vi "Read file.vi"(5 "Clk index":i32=1, 7 "Det index":i32, 8 "error in (no error)":errorcluster, 10 "Averaging range":dbl=1e-08 format="%#_13g", 11 "file (use dialog) in":path) -> (0 "Error Out":errorcluster, 1 "Polarity":enum16{"falling", "rising"}(ring), 2 "Waveform Array":waveform(dbl)[](array[waveform]), 3 "file (use dialog) out":path)   [LabVIEW 2020]
uses:
  <vilib>/Analysis/baseanly.llb/Mean (DBL).vi
  <vilib>/Utility/xml.llb/Read From XML File(array).vi
  <vilib>/Analysis/NI_AALBase.lvlib
panel:
  out "Running average (use odd integer)":i32=9
  out "XML Elements":string[](array[string])
  out "dt":dbl[](array[numeric])
  out "Ys":dbl[][](array[numeric])
  out "before substring":string
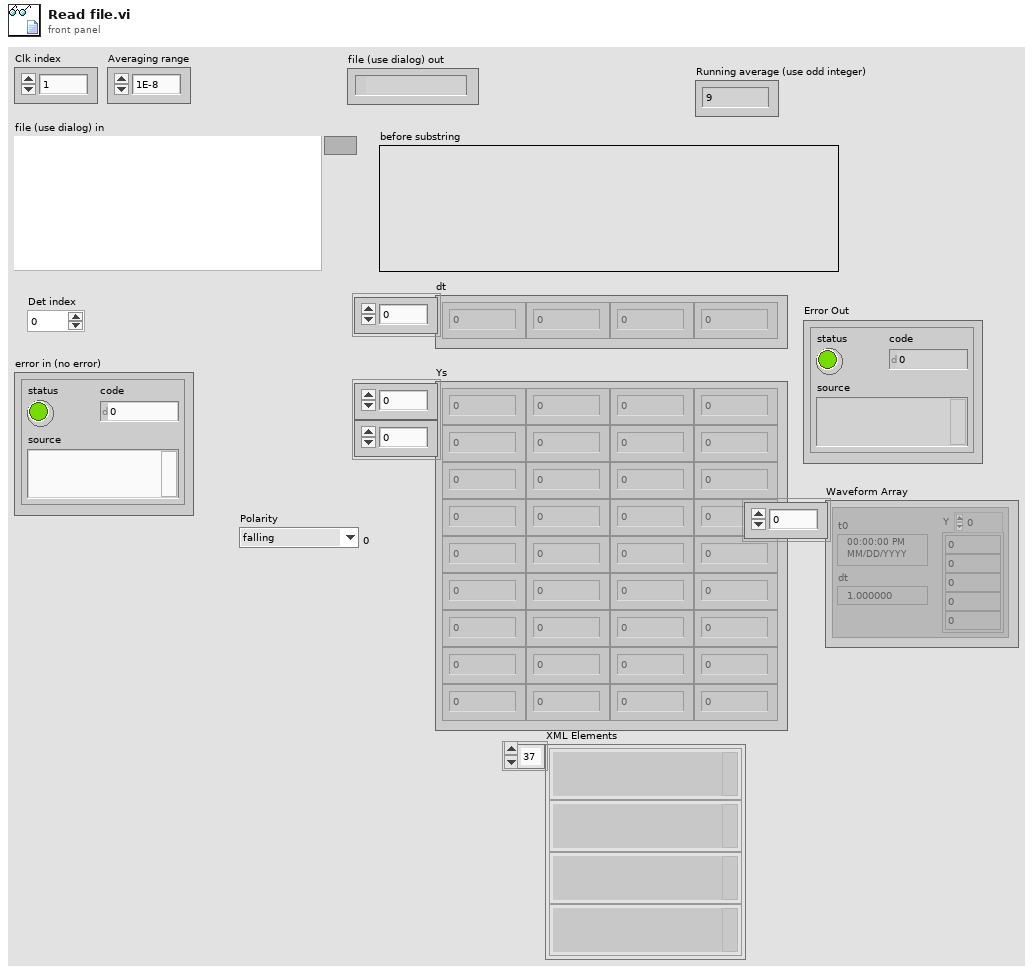
[diagram p1: front panel]
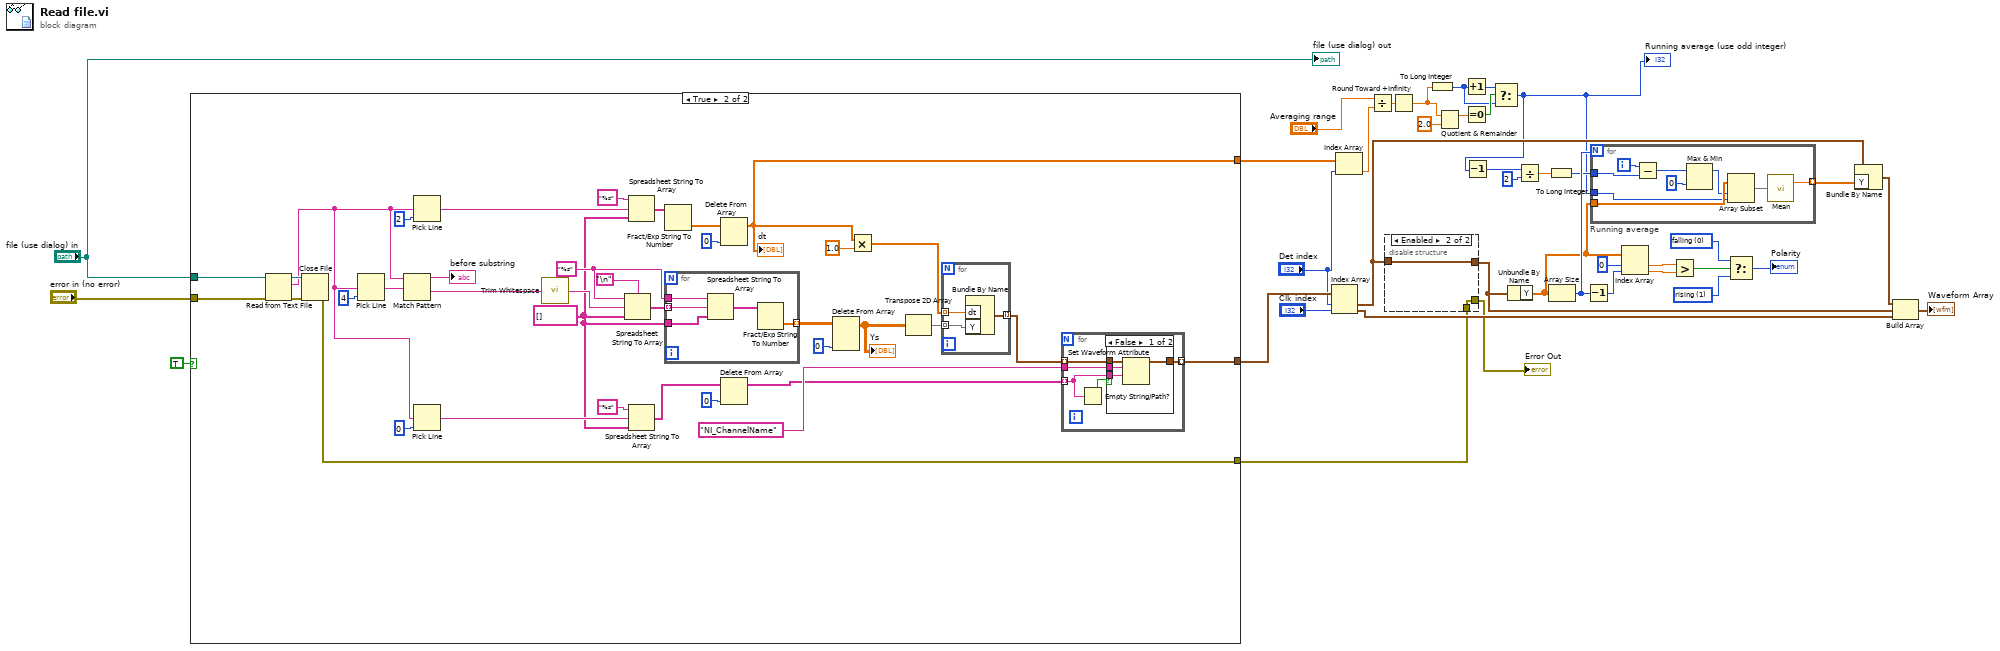
[diagram p0: block diagram]
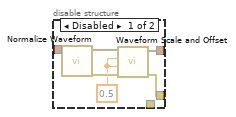
[diagram p2: hidden frame]
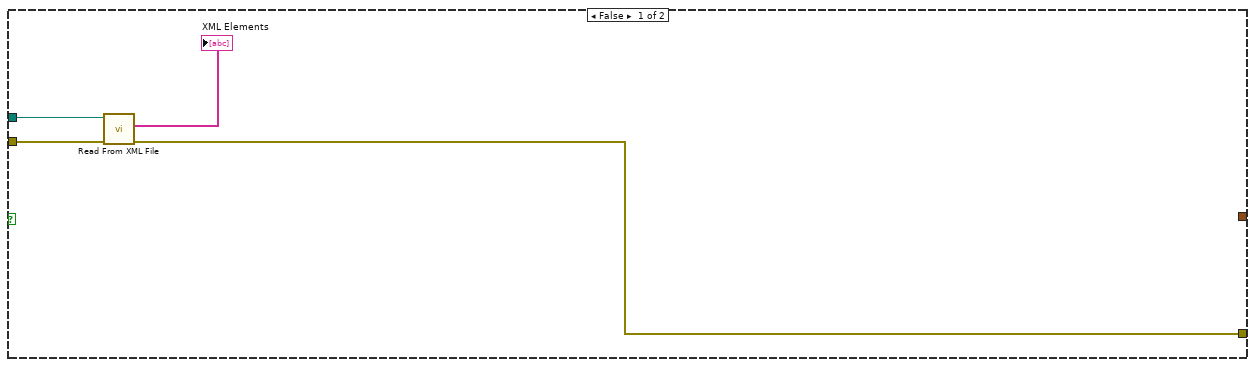
[diagram p3: hidden frame]
diagram:
  w30 = u16 1 items=["falling", "rising"] ("polarity (rising)")
  w31 = u16 0 items=["falling", "rising"] ("polarity (rising)")
  n1 = case shown="True" TRUE {
    tunnel: [_ w80] -> w32
    tunnel: "file (use dialog) in" -> [w42 w79]
    tunnel: "error in (no error)" -> [w43 w78]
    tunnel: [_ w45] -> w13
    tunnel: [w40 w44] -> w1
    frame False {
      n2 = call-poly <vilib>:"Read From XML File.vi"("error in (no error)"=w43, "XML File Path"=w42) -> ("error out"=w40:errorcluster, "XML Elements"=→"XML Elements":string[])  [unwired: 7 in, 1 out]
    }
    frame True {
      w68 = "%s" ("format string")
      w49 = string[] []
      n3 = Read from Text File(file (use dialog)=w79, error in=w78) -> (refnum out=w77:refnum<file>, text=w52:string, error out=w76:errorcluster)  [unwired: 2 in, 1 out]
      n4 = Close File(refnum=w77, error in=w76) -> (error out=w44:errorcluster)  [unwired: 1 out]
      n5 = Pick Line(multi-line string=w52, line index=4) -> (output string=w74:string)  [unwired: 1 in]
      n6 = Match Pattern(string=w52, regular expression=w74) -> (before substring=→"before substring":string, after substring=w60:string)  [unwired: 1 in, 2 out]
      n7 = Pick Line(multi-line string=w52, line index=2) -> (output string=w71:string)  [unwired: 1 in]
      n8 = Pick Line(multi-line string=w52, line index=0) -> (output string=w54:string)  [unwired: 1 in]
      n9 = call <vilib>:"Trim Whitespace.vi"("string"=w60) -> ("trimmed string"=w59:string)  [unwired: 1 in]
      n10 = Spreadsheet String To Array(delimiter (Tab)="\n", format string=w68, spreadsheet string=w59, array type (2D Dbl)=w49) -> (array=w70:string[])
      n11 = Spreadsheet String To Array(format string="%s", spreadsheet string=w71, array type (2D Dbl)=w49) -> (array=w64:string[])  [unwired: 1 in]
      n12 = Spreadsheet String To Array(format string="%s", spreadsheet string=w54, array type (2D Dbl)=w49) -> (array=w50:string[])  [unwired: 1 in]
      n13 = Fract/Exp String To Number(string=w64) -> (number=w63:dbl[])  [unwired: 3 in, 1 out]
      n14 = for {
        tunnel: w49 -> [w98]
        tunnel: w70 -> [w97] mode=indexing
        tunnel: [w95] -> w66 mode=indexing
        tunnel: w68 -> [w94]
        n15 = Spreadsheet String To Array(format string=w94, spreadsheet string=w97, array type (2D Dbl)=w98) -> (array=w96:string[])  [unwired: 1 in]
        n16 = Fract/Exp String To Number(string=w96) -> (number=w95:dbl[])  [unwired: 3 in, 1 out]
      }
      n17 = Delete From Array(array=w63, index=0 ("disabled index (col)")) -> (array with subset deleted=w45:dbl[])  [unwired: 1 in, 1 out]
      "dt" <- w45
      n18 = Delete From Array(array=w50, index=0 ("disabled index (col)")) -> (array with subset deleted=w48:string[])  [unwired: 1 in, 1 out]
      n19 = Delete From Array(array=w66, index (col)=0 ("disabled index (col)")) -> (array with subset deleted=w58:dbl[][])  [unwired: 2 in, 1 out]
      "Ys" <- w58
      n20 = Multiply(x=w45, y=1.0) -> (x*y=w46:dbl[])
      n21 = Transpose 2D Array(2D array=w58) -> (transposed array=w61:dbl[][])
      n22 = for {
        tunnel: w46 -> [w93] mode=indexing
        tunnel: w61 -> [w92] mode=indexing
        tunnel: [w91] -> w56 mode=indexing
        n23 = Bundle By Name("dt"=w93, "Y"=w92) -> (w91:waveform(dbl))  [unwired: 1 in]
      }
      n24 = for {
        tunnel: w56 -> [w85] mode=indexing
        tunnel: w48 -> [w82] mode=indexing
        tunnel: "NI_ChannelName" ("name") -> [w84]
        tunnel: [w83] -> w80 mode=indexing
        n25 = Empty String/Path?(string/path=w82) -> (empty?=w81:bool)
        n26 = case shown="False" w81 {
          tunnel: w85 -> [w89 w90]
          tunnel: w84 -> [w88 _]
          tunnel: [w87 w90] -> w83
          tunnel: w82 -> [w86 _]
          frame False {
            n27 = Set Waveform Attribute(5:w86, 6:w88, 7:w89) -> (3:w87:waveform(dbl))  [unwired: 1 in, 2 out]
          }
          frame True {
          }
        }
      }
    }
  }
  n28 = Index Array(array=w32, index #1="Det index", index #2="Clk index") -> (element #1=w15:waveform(dbl), element #2=w38:waveform(dbl))
  n29 = Index Array(array=w13, index="Det index") -> (element=w10:dbl)
  n30 = Divide(x="Averaging range", y=w10) -> (x/y=w5:dbl)
  n31 = disable-structure shown="Enabled" {
    disable-tunnel: [w103 w105] -> w17
    disable-tunnel: [w102 w106] -> w16
    disable-tunnel: w15 -> [w101 w106]
    disable-tunnel: w1 -> [_ w105]
    frame Disabled {
      w99 = 0.5 ("scale")
      n32 = call <vilib>:"Normalize Waveform.vi"("waveform in"=w101) -> ("error out"=w104:errorcluster, "normalized waveform"=w100:waveform(dbl))  [unwired: 7 in, 2 out]
      n33 = call <vilib>:"Waveform Scale and Offset.vi"("error in (no error)"=w104, "scale"=w99, "offset"=w99, "waveform in"=w100) -> ("error out"=w103:errorcluster, "waveform out"=w102:waveform(dbl))  [unwired: 6 in]
    }
    frame Enabled {
    }
  }
  "Error Out" <- w17
  n34 = Round Toward +Infinity(x=w5) -> (ceil(x): smallest int >= x=w4:dbl)
  n35 = To Long Integer(number=w4) -> (32bit integer=w3:i32)
  n36 = Quotient & Remainder(x=w4, y=2.0) -> (x-y*floor(x/y)=w6:dbl)  [unwired: 1 out]
  n37 = Increment(x=w3) -> (x+1=w7:i32)
  n38 = Equal To 0?(x=w6) -> (x = 0?=w8:bool)
  n39 = Select(t=w7, s=w8, f=w3) -> (s? t:f=w2:i32)
  "Running average (use odd integer)" <- w2
  n40 = Decrement(x=w2) -> (x-1=w14:i32)
  n41 = Unbundle By Name(w16) -> ("Y"=w25:dbl[])
  n42 = Divide(x=w14, y=2) -> (x/y=w23:dbl)
  n43 = To Long Integer(number=w23) -> (32bit integer=w24:i32)
  n44 = Array Size(array=w25) -> (size(s)=w35:i32)
  n45 = Decrement(x=w35) -> (x-1=w26:i32)
  n46 = for "Running average" {
    N: w35 -> [_]
    tunnel: w25 -> [w114]
    tunnel: [w115] -> w21 mode=indexing
    tunnel: w2 -> [w108]
    tunnel: w24 -> [w107]
    i -> [w112]
    n47 = Subtract(x=w112, y=w107) -> (x-y=w111:i32)
    n48 = Max & Min(x=w111, y=0) -> (max(x,y)=w109:i32)  [unwired: 1 out]
    n49 = Array Subset(array=w114, index=w109, length=w108) -> (w113:dbl[])
    n50 = call-poly <vilib>:"Mean.vi"("X"=w113) -> ("mean"=w115:dbl)  [unwired: 1 out]
  }
  n51 = Index Array(array=w25, index #1=0 ("index"), index #2=w26) -> (element #1=w28:dbl, element #2=w29:dbl)
  n52 = Greater?(x=w28, y=w29) -> (0:w34:bool)
  n53 = Select(t=w31, s=w34, f=w30) -> (s? t:f=→"Polarity":u16)
  n54 = Bundle By Name(cluster=w15, "Y"=w21) -> (w37:waveform(dbl))
  n55 = Build Array(w37, w16, w38) -> (→"Waveform Array":waveform(dbl)[])
  "file (use dialog) out" <- "file (use dialog) in"
